vi "DelayPlat3.vi"(8 "error In":errorcluster caption="error constant", 10 "DelayTime":u32, 11 "Bool":refnum<vi>) -> (0 "error Out":errorcluster caption="error constant")   [LabVIEW 2011]
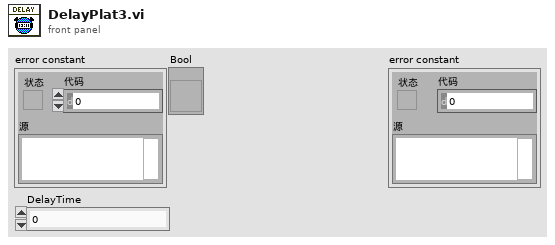
[diagram p1: front panel]
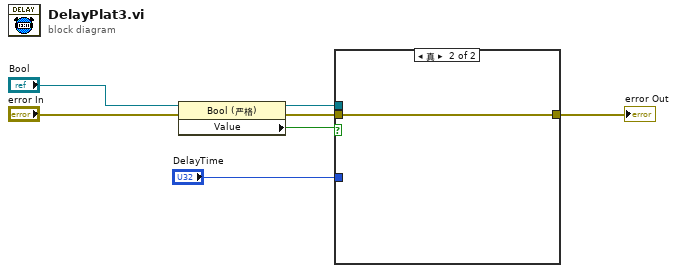
[diagram p0: block diagram]
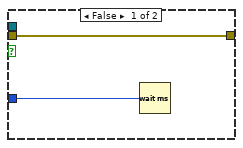
[diagram p2: hidden frame]
diagram:
  n1 = property class="Bool (严格)"(reference="Bool", error in="error In") -> (reference out=w4:refnum<vi>, error out=w3:errorcluster, "Value"=w5:bool)
  n2 = case shown="真" w5 {
    tunnel: w4 -> [_ _]
    tunnel: w3 -> [w9 w10]
    tunnel: [w9 w10] -> w2
    tunnel: "DelayTime" -> [w8 _]
    frame False {
      n3 = Wait (ms)(milliseconds to wait=w8) -> ()  [unwired: 1 out]
    }
    frame True {
    }
  }
  "error Out" <- w2
